vi "Teleop.vi"(10 "Match Info":T1={"Autonomous Elapsed Seconds"=0.0, "TeleOp Elapsed Seconds"=0.0, "Disabled Elapsed Seconds"=0.0, "Visited Autonomous"=FALSE, "Visited TeleOp"=FALSE, "Visited Disabled"=FALSE, "Autonomous Settings"={"Autonomous Style"=enum."Independent", "VI Refnum"=refnum}}, 11 "Call Context":T2) -> ()   [LabVIEW 2018]
doc: "This VI is called for each TeleOp packet received from the DS where the robot is not disabled. It is often used to read from the joysticks and update I/O or to update setpoints for timed control loops. It should complete and return within 20 milliseconds or it may miss DS packets."
uses:
  <vilib>/Rock Robotics/WPI/DriverStation/WPI_DriverStationDerivedRobotMode.ctl
  <vilib>/Rock Robotics/WPI/DriverStation/WPI_DriverStationMatch Info.ctl
  <vilib>/Rock Robotics/WPI/Utilities/WPI_GetSetVariantRefNum.vi
  Robot Global Data.vi
panel:
  out "Potentiometer":dbl
  out "Right Motor Speed":dbl
  out "Yaw":dbl
  out "Left Motor Speed":dbl
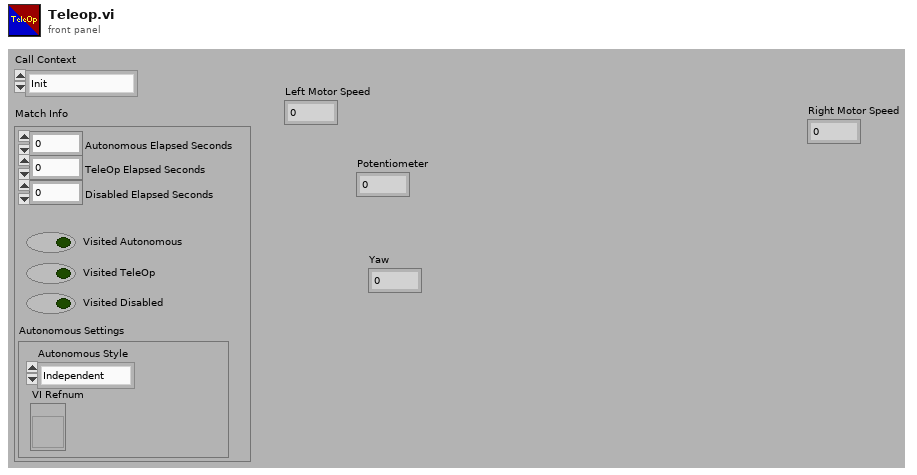
[diagram p1: front panel]
types:
  T1 = typedef "WPI_DriverStationMatch Info.ctl" = cluster{"Autonomous Elapsed Seconds":dbl, "TeleOp Elapsed Seconds":dbl, "Disabled Elapsed Seconds":dbl, "Visited Autonomous":bool, "Visited TeleOp":bool, "Visited Disabled":bool, "Autonomous Settings":cluster{"Autonomous Style":enum16{"Iterative", "Independent"}, "VI Refnum":refnum<vi>}}
  T2 = typedef "WPI_DriverStationDerivedRobotMode.ctl" = enum16{"Init", "Execute", "Stop"}
  T3 = typedef "WPI_JoystickDevRef.ctl" = cluster{"Device":T4}
  T4 = typedef "WPI_JoystickDeviceEnum.ctl" = enum16{"USB 0", "USB 1", "USB 2", "USB 3", "USB 4", "USB 5"}
  T5 = cluster{"Axes":dbl[], "Buttons":bool[], "POVs":i16[]}
  T6 = cluster{"Yaw":dbl, "Roll":dbl, "Pitch":dbl, "Heading":dbl, "Fused Heading":dbl}
  T7 = typedef "WPI_PotentiometerDevRef.ctl" = cluster{"DevStatus":errorcluster, "Analog Channel":T8, "Invert Output":bool}
  T8 = typedef "FPGA_AIChannel.ctl" = enum8{"AI 0", "AI 1", "AI 2", "AI 3", "AI MXP 0", "AI MXP 1", "AI MXP 2", "AI MXP 3", "Invalid"}
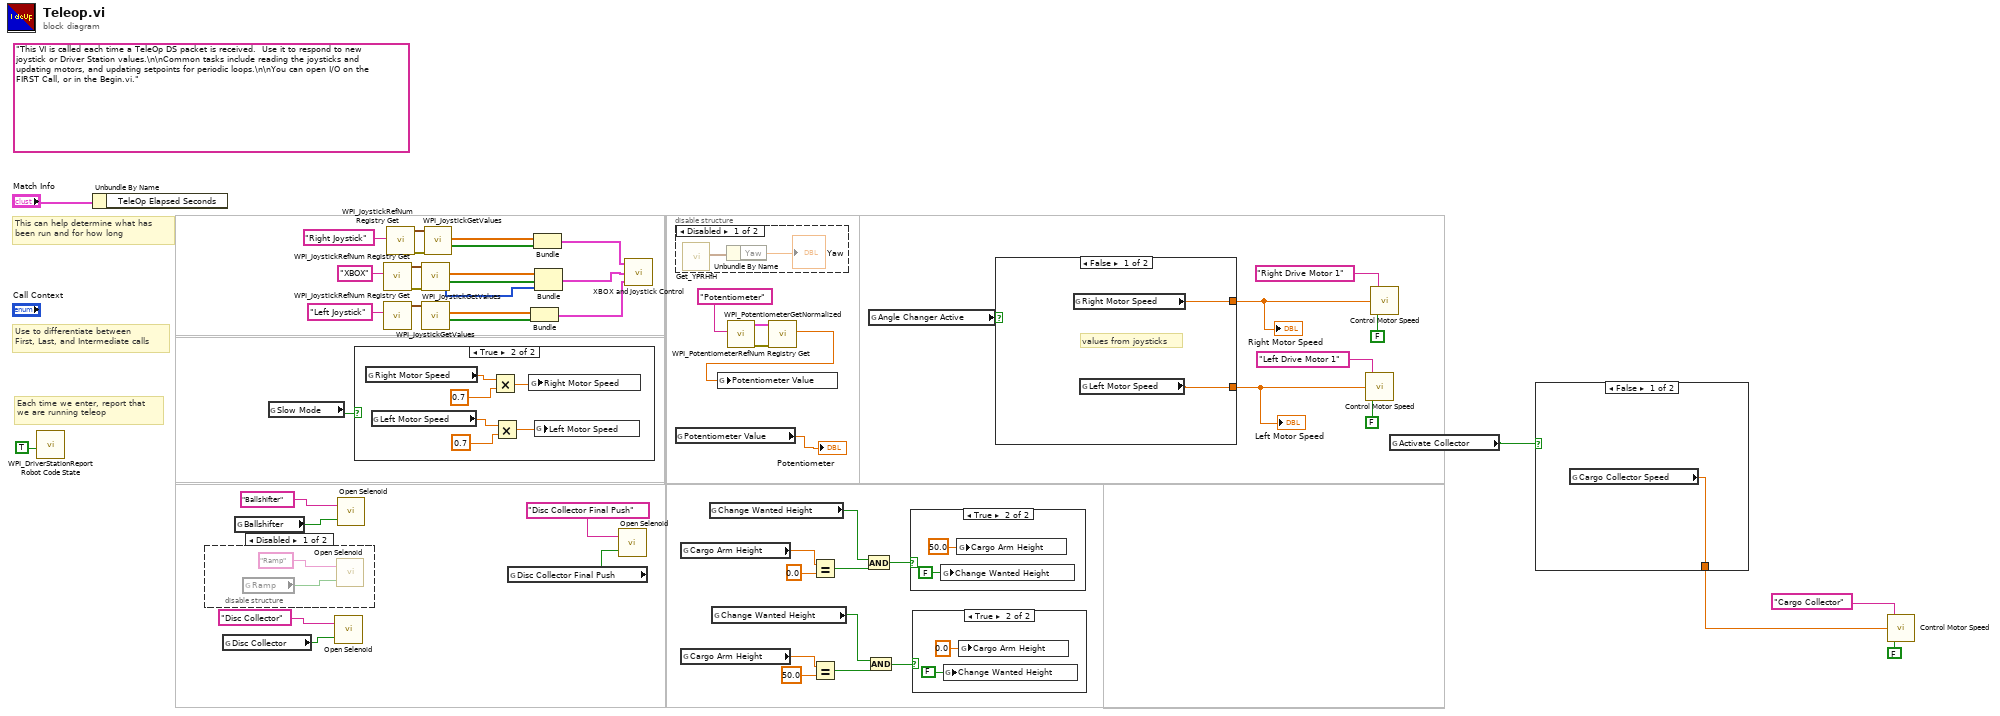
[diagram p0: block diagram]
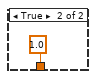
[diagram p2: hidden frame]
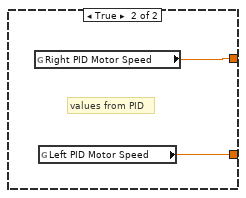
[diagram p4: hidden frame]
diagram:
  (unwired) "This VI is called each time a TeleOp DS packet is received.  Use it to respond to new joystick or Driver Station values.\n\nCommon tasks include reading the joysticks and updating motors, and updating setpoints for periodic loops.\n\nYou can open I/O on the FIRST Call, or in the Begin.vi."
  # "Each time we enter, report that\nwe are running teleop"
  # "Use to differentiate between\nFirst, Last, and Intermediate calls"
  # "This can help determine what has\nbeen run and for how long"
  n1 = call <vilib>:"WPI_DriverStationReport Robot Code State.vi"("TeleOp"=TRUE ("Autonomous")) -> ()  [unwired: 10 in, 1 out]
  n2 = Unbundle By Name("Match Info") -> ()  [unwired: 1 out]
  n3 = disable-structure shown="Disabled" {
    frame Disabled {
      n4 = global read "Robot Global Data.vi" "Ramp"() -> (w54:bool)
      n5 = call "Open Selenoid.vi"("Enable"=w54, "Selenoid Name"="Ramp") -> ()  [unwired: 1 in]
    }
    frame Enabled {
    }
  }
  n6 = global read "Robot Global Data.vi" "Disc Collector"() -> (w30:bool)
  n7 = global read "Robot Global Data.vi" "Ballshifter"() -> (w32:bool)
  n8 = global read "Robot Global Data.vi" "Slow Mode"() -> (w13:bool)
  n9 = call "Open Selenoid.vi"("Enable"=w30, "Selenoid Name"="Disc Collector") -> ()  [unwired: 1 in]
  n10 = call "Open Selenoid.vi"("Enable"=w32, "Selenoid Name"="Ballshifter") -> ()  [unwired: 1 in]
  n11 = case shown="True" w13 {
    frame False {
    }
    frame True {
      n12 = global read "Robot Global Data.vi" "Right Motor Speed"() -> (w60:dbl)
      n13 = global read "Robot Global Data.vi" "Left Motor Speed"() -> (w57:dbl)
      n14 = Multiply(x=w60, y=0.7) -> (x*y=w59:dbl)
      n15 = Multiply(x=w57, y=0.7) -> (x*y=w56:dbl)
      n16 = global write "Robot Global Data.vi" "Right Motor Speed"(w59) -> ()
      n17 = global write "Robot Global Data.vi" "Left Motor Speed"(w56) -> ()
    }
  }
  n18 = call <vilib>:"WPI_JoystickRefNum Registry Get.vi"("refnum name"="XBOX") -> ("error out"=w51:errorcluster, "JoystickDevRef"=w50:T3)  [unwired: 9 in]
  n19 = call <vilib>:"WPI_JoystickRefNum Registry Get.vi"("refnum name"="Left Joystick") -> ("JoystickDevRef"=w45:T3)  [unwired: 9 in, 1 out]
  n20 = call <vilib>:"WPI_JoystickRefNum Registry Get.vi"("refnum name"="Right Joystick") -> ("error out"=w48:errorcluster, "JoystickDevRef"=w47:T3)  [unwired: 9 in]
  n21 = call <vilib>:"WPI_JoystickGetValues.vi"("error in (no error)"=w51, "JoystickDevRef"=w50) -> ("Buttons"=w40:bool[], "Axes"=w41:dbl[], "POVs"=w9:i16[])  [unwired: 5 in, 2 out]
  n22 = call <vilib>:"WPI_JoystickGetValues.vi"("JoystickDevRef"=w45) -> ("Buttons"=w38:bool[], "Axes"=w42:dbl[])  [unwired: 6 in, 3 out]
  n23 = call <vilib>:"WPI_JoystickGetValues.vi"("error in (no error)"=w48, "JoystickDevRef"=w47) -> ("Buttons"=w43:bool[], "Axes"=w39:dbl[])  [unwired: 5 in, 3 out]
  n24 = global read "Robot Global Data.vi" "Disc Collector Final Push"() -> (w16:bool)
  n25 = Bundle("Axes"=w42, "Buttons"=w38) -> (w36:cluster{"Axes":dbl[], "Buttons":bool[]})  [unwired: 1 in]
  n26 = Bundle("Axes"=w39, "Buttons"=w43) -> (w37:cluster{"Axes":dbl[], "Buttons":bool[]})  [unwired: 1 in]
  n27 = Bundle("Axes"=w41, "Buttons"=w40, "POVs"=w9) -> (w8:T5)  [unwired: 1 in]
  n28 = call "Open Selenoid.vi"("Enable"=w16, "Selenoid Name"="Disc Collector Final Push") -> ()  [unwired: 1 in]
  n29 = call "XBOX and Joystick Control.vi"("Left Joystick"=w36, "XBOX"=w8, "Right Joystick"=w37) -> ()  [unwired: 1 in]
  n30 = disable-structure shown="Disabled" {
    frame Disabled {
      n31 = call <vilib>:"Get_YPRHfH.vi"() -> ("YRPHfH"=w63:T6)  [unwired: 11 in]
      n32 = Unbundle By Name(w63) -> ("Yaw"=→"Yaw":dbl)
    }
    frame Enabled {
    }
  }
  n33 = global read "Robot Global Data.vi" "Potentiometer Value"() -> (→"Potentiometer":dbl)
  n34 = global read "Robot Global Data.vi" "Cargo Arm Height"() -> (w27:dbl)
  n35 = global read "Robot Global Data.vi" "Cargo Arm Height"() -> (w22:dbl)
  n36 = global read "Robot Global Data.vi" "Change Wanted Height"() -> (w24:bool)
  n37 = global read "Robot Global Data.vi" "Change Wanted Height"() -> (w19:bool)
  n38 = call <vilib>:"WPI_PotentiometerRefNum Registry Get.vi"("refnum name"="Potentiometer") -> ("error out"=w7:errorcluster, "PotDevRef"=w6:T7)  [unwired: 9 in]
  n39 = call <vilib>:"WPI_PotentiometerGetNormalized.vi"("error in"=w7, "PotDevRef"=w6) -> ("Normalized Value"=w5:dbl)  [unwired: 7 in, 2 out]
  n40 = global write "Robot Global Data.vi" "Potentiometer Value"(w5) -> ()
  n41 = Equal?(x=w27, y=0.0) -> (x = y?=w25:bool)
  n42 = Equal?(x=w22, y=50.0) -> (x = y?=w20:bool)
  n43 = And(x=w24, y=w25) -> (x .and. y?=w23:bool)
  n44 = And(x=w19, y=w20) -> (x .and. y?=w18:bool)
  n45 = global read "Robot Global Data.vi" "Angle Changer Active"() -> (w10:bool)
  n46 = case shown="True" w23 {
    frame False {
    }
    frame True {
      n47 = global write "Robot Global Data.vi" "Change Wanted Height"(FALSE ("Change Wanted Height")) -> ()
      n48 = global write "Robot Global Data.vi" "Cargo Arm Height"(50.0 ("Cargo Arm Height")) -> ()
    }
  }
  n49 = case shown="True" w18 {
    frame False {
    }
    frame True {
      n50 = global write "Robot Global Data.vi" "Change Wanted Height"(FALSE ("Change Wanted Height")) -> ()
      n51 = global write "Robot Global Data.vi" "Cargo Arm Height"(0.0 ("Cargo Arm Height")) -> ()
    }
  }
  n52 = case shown="False" w10 {
    tunnel: [w69 w71] -> w12
    tunnel: [w68 w70] -> w11
    frame False {
      # "values from joysticks"
      n53 = global read "Robot Global Data.vi" "Right Motor Speed"() -> (w69:dbl)
      n54 = global read "Robot Global Data.vi" "Left Motor Speed"() -> (w68:dbl)
    }
    frame True {
      # "values from PID"
      n55 = global read "Robot Global Data.vi" "Right PID Motor Speed"() -> (w71:dbl)
      n56 = global read "Robot Global Data.vi" "Left PID Motor Speed"() -> (w70:dbl)
    }
  }
  "Left Motor Speed" <- w11
  "Right Motor Speed" <- w12
  n57 = call "Control Motor Speed.vi"("Invert"=FALSE, "Speed"=w11, "Motor Name"="Left Drive Motor 1") -> ()  [unwired: 1 in]
  n58 = call "Control Motor Speed.vi"("Invert"=FALSE, "Speed"=w12, "Motor Name"="Right Drive Motor 1") -> ()  [unwired: 1 in]
  n59 = global read "Robot Global Data.vi" "Activate Collector"() -> (w2:bool)
  n60 = case shown="False" w2 {
    tunnel: [w72 1.0 ("Cargo Collector Speed")] -> w1
    frame False {
      n61 = global read "Robot Global Data.vi" "Cargo Collector Speed"() -> (w72:dbl)
    }
    frame True {
    }
  }
  n62 = call "Control Motor Speed.vi"("Invert"=FALSE, "Speed"=w1, "Motor Name"="Cargo Collector") -> ()  [unwired: 1 in]
